vi "Finish.vi"   [LabVIEW 2014]
doc: "This VI is called just before exiting. It is expected to close I/O refnum, save collected data, etc."
uses:
  <vilib>/Rock Robotics/WPI/Joystick/WPI_JoystickGetSetRefNum.vi
  <vilib>/Rock Robotics/WPI/RobotDrive/WPI_RobotDriveGetSetRefNum.vi
types:
  T1 = typedef "WPI_DigitalInputDevRef.ctl" = cluster{"DevStatus":errorcluster, "DIO Channel":T2, "Controller":T3}
  T2 = typedef "FPGA_DIOChannel.ctl" = enum8{"DIO 0", "DIO 1", "DIO 2", "DIO 3", "DIO 4", "DIO 5", "DIO 6", "DIO 7", "DIO 8", "DIO 9", "DIO MXP 0", "DIO MXP 1", "DIO MXP 2", "DIO MXP 3", "DIO MXP 4", "DIO MXP 5", "DIO MXP 6", "DIO MXP 7", "DIO MXP 8", "DIO MXP 9", "DIO MXP 10", "DIO MXP 11", "DIO MXP 12", "DIO MXP 13", "DIO MXP 14", "DIO MXP 15", "Invalid"}
  T3 = typedef "FPGA_TypedefDigitalModule.ctl" = enum16{"Controller 1"}
  T4 = typedef "WPI_AnalogChannelDevRef.ctl" = cluster{"DevStatus":errorcluster, "Controller":T5, "Analog Channel":T6}
  T5 = typedef "FPGA_TypedefAnalogModule.ctl" = enum16{"Controller 1"}
  T6 = typedef "FPGA_AIChannel.ctl" = enum8{"AI 0", "AI 1", "AI 2", "AI 3", "AI MXP 0", "AI MXP 1", "AI MXP 2", "AI MXP 3", "Invalid"}
  T7 = typedef "WPI_DigitalOutputDevRef.ctl" = cluster{"Controller":T3, "DIO Channel":T2, "DevStatus":errorcluster}
  T8 = typedef "WPI_GyroDevRef.ctl" = cluster{"DevStatus":errorcluster, "Analog Module":T5, "Analog Channel":T6, "Offset":dbl, "Gain (VoltsPerDegree/Second)":dbl}
  T9 = typedef "WPI_EncoderDevRef.ctl" = cluster{"DevStatus":errorcluster, "EncoderIndex":T10, "CounterIndex":T11, "DistancePerCount":dbl, "Decoding Type":T12}
  T10 = typedef "FPGA_EncoderIdx.ctl" = enum8{"Enc 0", "Enc 1", "Enc 2", "Enc 3", "Enc 4", "Enc 5", "Enc 6", "Enc 7", "Invalid"}
  T11 = typedef "FPGA_CounterCtrSystemIndex.ctl" = enum8{"Ctr 0", "Ctr 1", "Ctr 2", "Ctr 3", "Ctr 4", "Ctr 5", "Ctr 6", "Ctr 7", "Invalid"}
  T12 = typedef "WPI_EncoderType.ctl" = enum16{"1x", "2x", "4x"}
  T13 = typedef "WPI_MotorControlDeviceRef.ctl" = cluster{"DeviceStatus":errorcluster, "Type":T14, "PWM":cluster{"Controller":T3, "PWM Channel":T15, "DeadBand":T16}, "CAN":cluster{"Device Number":u8, "Control Mode":T17, "Semaphore":T18, "Max Vout":dbl, "TalonSRX Control Mode":T19}, "Invert":bool, "TransformRef":T20, "InvTransformRef":T20}
  T14 = typedef "WPI_MotorControlType.ctl" = enum16{"PWM", "CAN", "CANTalonSRX"}
  T15 = typedef "FPGA_DIOPWMChannel.ctl" = enum8{"PWM 0", "PWM 1", "PWM 2", "PWM 3", "PWM 4", "PWM 5", "PWM 6", "PWM 7", "PWM 8", "PWM 9", "PWM MXP 0", "PWM MXP 1", "PWM MXP 2", "PWM MXP 3", "PWM MXP 4", "PWM MXP 5", "PWM MXP 6", "PWM MXP 7", "PWM MXP 8", "PWM MXP 9", "Invalid"}
  T16 = typedef "WPI_PWMDeadband.ctl" = cluster{"Name":string, "maxPositivePwm":i32, "minPositivePwm":i32, "centerPwm":i32, "maxNegativePwm":i32, "minNegativePwm":i32, "angularRange":u16}
  T17 = typedef "WPI_CANJaguar_ControlMode.ctl" = enum8{"Percent VBus", "Current", "Speed", "Position", "Voltage"}
  T18 = typedef "Semaphore RefNum" = refnum<k1>
  T19 = typedef "WPI_CANTalonSRX_APIControlMode.ctl" = enum8{"Percent VBus", "Speed", "Position", "Slave", "Unchanged / Invalid"}
  T20 = typedef "WPI_PWMTransform_ConPane.ctl" = refnum<vi>
  T21 = typedef "WPI_JoystickDevRef.ctl" = cluster{"Device":T22}
  T22 = typedef "WPI_JoystickDeviceEnum.ctl" = enum16{"USB 0", "USB 1", "USB 2", "USB 3", "USB 4", "USB 5"}
  T23 = typedef "WPI_RobotDriveDevRef.ctl" = cluster{"DevStatus":errorcluster, "Motors[]":T13[], "Square Inputs":bool, "Max Output":dbl}
  T24 = typedef "WPI_SolenoidDevRef.ctl" = cluster{"DevStatus":errorcluster, "Pneumatics Control Module":u8, "Forward Solenoid Channel":T25, "Reverse Solenoid Channel":T25}
  T25 = typedef "WPI_SolenoidChannel.ctl" = enum8{"Solenoid 0", "Solenoid 1", "Solenoid 2", "Solenoid 3", "Solenoid 4", "Solenoid 5", "Solenoid 6", "Solenoid 7", "Invalid"}
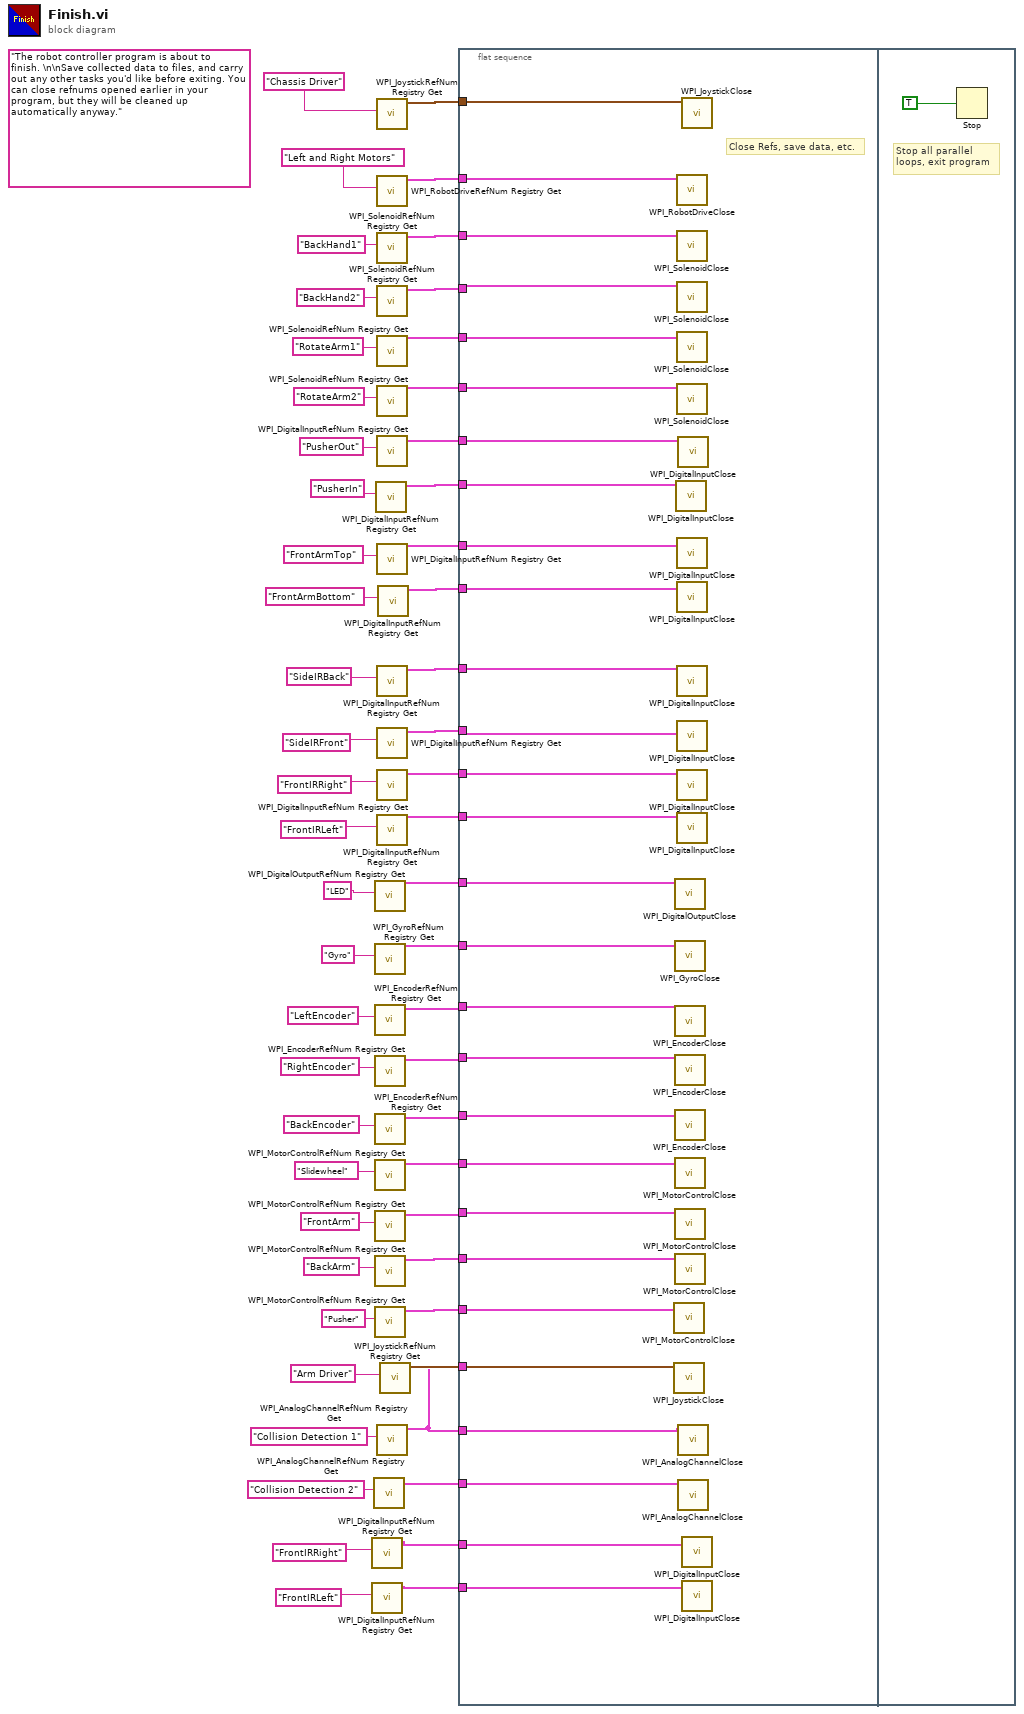
[diagram p0: block diagram]
diagram:
  (unwired) "The robot controller program is about to finish. \n\nSave collected data to files, and carry out any other tasks you'd like before exiting. You can close refnums opened earlier in your program, but they will be cleaned up automatically anyway."
  n1 = call <vilib>:"WPI_DigitalInputRefNum Registry Get.vi"("refnum name"="FrontIRRight") -> ("DigitalInputDevRef"=w1:T1)  [unwired: 9 in, 1 out]
  n2 = call <vilib>:"WPI_DigitalInputRefNum Registry Get.vi"("refnum name"="FrontIRLeft") -> ("DigitalInputDevRef"=w2:T1)  [unwired: 9 in, 1 out]
  n3 = call <vilib>:"WPI_AnalogChannelRefNum Registry Get.vi"("refnum name"="Collision Detection 2") -> ("AIDeviceRef"=w5:T4)  [unwired: 9 in, 1 out]
  n4 = call <vilib>:"WPI_DigitalOutputRefNum Registry Get.vi"("refnum name"="LED") -> ("DigitalOutputDevRef"=w43:T7)  [unwired: 9 in, 1 out]
  n5 = call <vilib>:"WPI_GyroRefNum Registry Get.vi"("refnum name"="Gyro") -> ("GyroDevRef"=w41:T8)  [unwired: 9 in, 1 out]
  n6 = call <vilib>:"WPI_EncoderRefNum Registry Get.vi"("refnum name"="LeftEncoder") -> ("EncoderDevRef"=w37:T9)  [unwired: 9 in, 1 out]
  n7 = call <vilib>:"WPI_EncoderRefNum Registry Get.vi"("refnum name"="RightEncoder") -> ("EncoderDevRef"=w38:T9)  [unwired: 9 in, 1 out]
  n8 = call <vilib>:"WPI_EncoderRefNum Registry Get.vi"("refnum name"="BackEncoder") -> ("EncoderDevRef"=w29:T9)  [unwired: 9 in, 1 out]
  n9 = call <vilib>:"WPI_MotorControlRefNum Registry Get.vi"("refnum name"="Slidewheel") -> ("MotorControlDevRef"=w34:T13)  [unwired: 9 in, 1 out]
  n10 = call <vilib>:"WPI_MotorControlRefNum Registry Get.vi"("refnum name"="FrontArm") -> ("MotorControlDevRef"=w35:T13)  [unwired: 9 in, 1 out]
  n11 = call <vilib>:"WPI_MotorControlRefNum Registry Get.vi"("refnum name"="BackArm") -> ("MotorControlDevRef"=w36:T13)  [unwired: 9 in, 1 out]
  n12 = call <vilib>:"WPI_MotorControlRefNum Registry Get.vi"("refnum name"="Pusher") -> ("MotorControlDevRef"=w24:T13)  [unwired: 9 in, 1 out]
  n13 = call <vilib>:"WPI_DigitalInputRefNum Registry Get.vi"("refnum name"="PusherIn") -> ("DigitalInputDevRef"=w18:T1)  [unwired: 9 in, 1 out]
  n14 = call <vilib>:"WPI_JoystickRefNum Registry Get.vi"("refnum name"="Chassis Driver") -> ("JoystickDevRef"=w53:T21)  [unwired: 1 in, 9 out]
  n15 = call <vilib>:"WPI_RobotDriveRefNum Registry Get.vi"("refnum name"="Left and Right Motors") -> ("RobotDriveDevRef"=w54:T23)  [unwired: 1 in, 9 out]
  n16 = call <vilib>:"WPI_SolenoidRefNum Registry Get.vi"("refnum name"="BackHand1") -> ("SolenoidDevRef"=w45:T24)  [unwired: 9 in, 1 out]
  n17 = call <vilib>:"WPI_SolenoidRefNum Registry Get.vi"("refnum name"="BackHand2") -> ("SolenoidDevRef"=w46:T24)  [unwired: 9 in, 1 out]
  n18 = call <vilib>:"WPI_SolenoidRefNum Registry Get.vi"("refnum name"="RotateArm1") -> ("SolenoidDevRef"=w47:T24)  [unwired: 9 in, 1 out]
  n19 = call <vilib>:"WPI_SolenoidRefNum Registry Get.vi"("refnum name"="RotateArm2") -> ("SolenoidDevRef"=w48:T24)  [unwired: 9 in, 1 out]
  n20 = call <vilib>:"WPI_DigitalInputRefNum Registry Get.vi"("refnum name"="PusherOut") -> ("DigitalInputDevRef"=w17:T1)  [unwired: 9 in, 1 out]
  n21 = call <vilib>:"WPI_DigitalInputRefNum Registry Get.vi"("refnum name"="FrontArmTop") -> ("DigitalInputDevRef"=w27:T1)  [unwired: 9 in, 1 out]
  n22 = call <vilib>:"WPI_DigitalInputRefNum Registry Get.vi"("refnum name"="SideIRBack") -> ("DigitalInputDevRef"=w11:T1)  [unwired: 9 in, 1 out]
  n23 = call <vilib>:"WPI_DigitalInputRefNum Registry Get.vi"("refnum name"="SideIRFront") -> ("DigitalInputDevRef"=w10:T1)  [unwired: 9 in, 1 out]
  n24 = call <vilib>:"WPI_DigitalInputRefNum Registry Get.vi"("refnum name"="FrontIRRight") -> ("DigitalInputDevRef"=w9:T1)  [unwired: 9 in, 1 out]
  n25 = call <vilib>:"WPI_DigitalInputRefNum Registry Get.vi"("refnum name"="FrontIRLeft") -> ("DigitalInputDevRef"=w8:T1)  [unwired: 9 in, 1 out]
  n26 = call <vilib>:"WPI_AnalogChannelRefNum Registry Get.vi"("refnum name"="Collision Detection 1") -> ("AIDeviceRef"=w7:T4)  [unwired: 9 in, 1 out]
  n27 = call <vilib>:"WPI_DigitalInputRefNum Registry Get.vi"("refnum name"="FrontArmBottom") -> ("DigitalInputDevRef"=w25:T1)  [unwired: 9 in, 1 out]
  n28 = call <vilib>:"WPI_JoystickRefNum Registry Get.vi"("refnum name"="Arm Driver") -> ("JoystickDevRef"=w21:T21)  [unwired: 1 in, 9 out]
  n29 = flat-sequence {
    tunnel: w54 -> [w84]
    tunnel: w53 -> [w83]
    tunnel: w48 -> [w82]
    tunnel: w47 -> [w81]
    tunnel: w46 -> [w80]
    tunnel: w45 -> [w79]
    tunnel: w43 -> [w78]
    tunnel: w41 -> [w77]
    tunnel: w38 -> [w76]
    tunnel: w37 -> [w75]
    tunnel: w36 -> [w74]
    tunnel: w35 -> [w73]
    tunnel: w34 -> [w72]
    tunnel: w29 -> [w71]
    tunnel: w27 -> [w70]
    tunnel: w25 -> [w69]
    tunnel: w24 -> [w68]
    tunnel: w21 -> [w67]
    tunnel: w18 -> [w66]
    tunnel: w17 -> [w65]
    tunnel: w7 -> [_]
    tunnel: w11 -> [w64]
    tunnel: w10 -> [w63]
    tunnel: w9 -> [w62]
    tunnel: w8 -> [w61]
    tunnel: w7 -> [w60]
    tunnel: w5 -> [w59]
    tunnel: w2 -> [w58]
    tunnel: w1 -> [w57]
    frame #0 {
      # "Close Refs, save data, etc."
      n30 = call <vilib>:"WPI_MotorControlClose.vi"("MotorControlDevRef"=w68) -> ()  [unwired: 10 in, 1 out]
      n31 = call <vilib>:"WPI_JoystickClose.vi"("JoystickDevRef"=w67) -> ()  [unwired: 11 out]
      n32 = call <vilib>:"WPI_DigitalOutputClose.vi"("DigitalOutputDevRef"=w78) -> ()  [unwired: 10 in, 1 out]
      n33 = call <vilib>:"WPI_GyroClose.vi"("GyroDevRef"=w77) -> ()  [unwired: 10 in, 1 out]
      n34 = call <vilib>:"WPI_EncoderClose.vi"("EncoderDevRef"=w75) -> ()  [unwired: 10 in, 1 out]
      n35 = call <vilib>:"WPI_EncoderClose.vi"("EncoderDevRef"=w76) -> ()  [unwired: 10 in, 1 out]
      n36 = call <vilib>:"WPI_EncoderClose.vi"("EncoderDevRef"=w71) -> ()  [unwired: 10 in, 1 out]
      n37 = call <vilib>:"WPI_MotorControlClose.vi"("MotorControlDevRef"=w72) -> ()  [unwired: 10 in, 1 out]
      n38 = call <vilib>:"WPI_MotorControlClose.vi"("MotorControlDevRef"=w73) -> ()  [unwired: 10 in, 1 out]
      n39 = call <vilib>:"WPI_MotorControlClose.vi"("MotorControlDevRef"=w74) -> ()  [unwired: 10 in, 1 out]
      n40 = call <vilib>:"WPI_DigitalInputClose.vi"("DigitalInputDevRef"=w66) -> ()  [unwired: 10 in, 1 out]
      n41 = call <vilib>:"WPI_RobotDriveClose.vi"("RobotDriveDevRef"=w84) -> ()  [unwired: 1 in, 10 out]
      n42 = call <vilib>:"WPI_SolenoidClose.vi"("SolenoidDevRef"=w79) -> ()  [unwired: 10 in, 1 out]
      n43 = call <vilib>:"WPI_SolenoidClose.vi"("SolenoidDevRef"=w80) -> ()  [unwired: 10 in, 1 out]
      n44 = call <vilib>:"WPI_SolenoidClose.vi"("SolenoidDevRef"=w81) -> ()  [unwired: 10 in, 1 out]
      n45 = call <vilib>:"WPI_SolenoidClose.vi"("SolenoidDevRef"=w82) -> ()  [unwired: 10 in, 1 out]
      n46 = call <vilib>:"WPI_DigitalInputClose.vi"("DigitalInputDevRef"=w70) -> ()  [unwired: 10 in, 1 out]
      n47 = call <vilib>:"WPI_DigitalInputClose.vi"("DigitalInputDevRef"=w69) -> ()  [unwired: 10 in, 1 out]
      n48 = call <vilib>:"WPI_DigitalInputClose.vi"("DigitalInputDevRef"=w64) -> ()  [unwired: 10 in, 1 out]
      n49 = call <vilib>:"WPI_DigitalInputClose.vi"("DigitalInputDevRef"=w63) -> ()  [unwired: 10 in, 1 out]
      n50 = call <vilib>:"WPI_DigitalInputClose.vi"("DigitalInputDevRef"=w62) -> ()  [unwired: 10 in, 1 out]
      n51 = call <vilib>:"WPI_DigitalInputClose.vi"("DigitalInputDevRef"=w61) -> ()  [unwired: 10 in, 1 out]
      n52 = call <vilib>:"WPI_DigitalInputClose.vi"("DigitalInputDevRef"=w65) -> ()  [unwired: 10 in, 1 out]
      n53 = call <vilib>:"WPI_AnalogChannelClose.vi"("AIDeviceRef"=w60) -> ()  [unwired: 10 in, 1 out]
      n54 = call <vilib>:"WPI_AnalogChannelClose.vi"("AIDeviceRef"=w59) -> ()  [unwired: 10 in, 1 out]
      n55 = call <vilib>:"WPI_JoystickClose.vi"("JoystickDevRef"=w83) -> ()  [unwired: 11 out]
      n56 = call <vilib>:"WPI_DigitalInputClose.vi"("DigitalInputDevRef"=w57) -> ()  [unwired: 10 in, 1 out]
      n57 = call <vilib>:"WPI_DigitalInputClose.vi"("DigitalInputDevRef"=w58) -> ()  [unwired: 10 in, 1 out]
    }
    frame #1 {
      # "Stop all parallel\nloops, exit program"
      n58 = Stop(stop? (T)=TRUE ("Quit")) -> ()
    }
  }
